vi "FPGA_SystemAsync VI Agent.vi"() -> ()   [LabVIEW 2017]
uses:
  <vilib>/Rock Robotics/SystemInterfaces/System/FPGA_SystemFPGA Ref Global.vi
panel:
  in  "Main Name":string
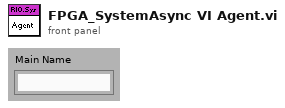
[diagram p1: front panel]
types:
  T1 = typedef "FPGA_SystemFRC FPGA Ref.ctl" = refnum<k20>
  T2 = enum32{"Bad", "Idle", "Run top level", "Running"}
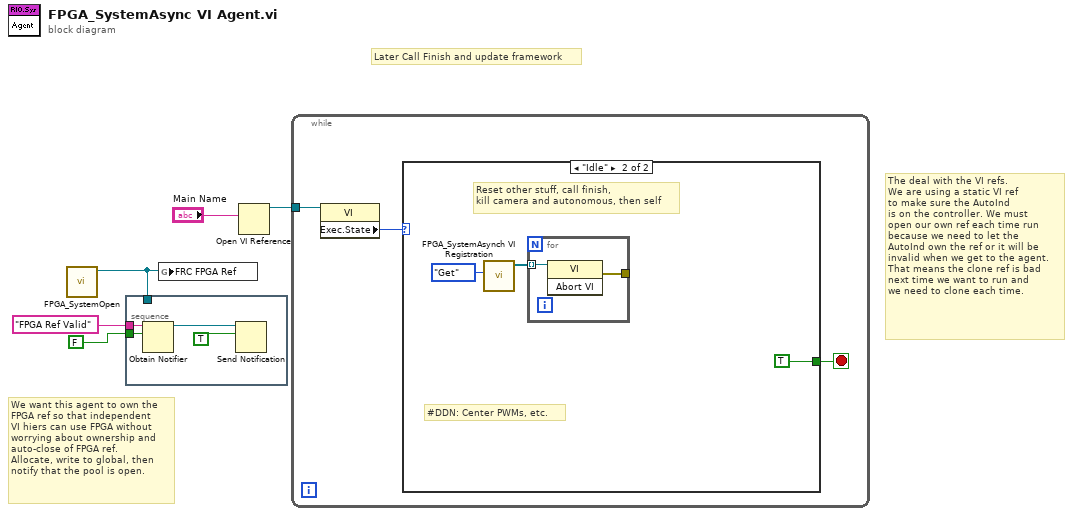
[diagram p0: block diagram]
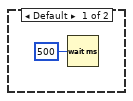
[diagram p2: hidden frame]
diagram:
  # "The deal with the VI refs.\nWe are using a static VI ref\nto make sure the AutoInd\nis on the controller. We must\nopen our own ref each time run\nbecause we need to let the\nAutoInd own the ref or it will be\ninvalid when we get to the agent.\nThat means the clone ref is bad\nnext time we want to run and\nwe need to clone each time."
  # "Later Call Finish and update framework"
  # "We want this agent to own the\nFPGA ref so that independent\nVI hiers can use FPGA without\nworrying about ownership and\nauto-close of FPGA ref.\nAllocate, write to global, then\nnotify that the pool is open."
  n1 = call <vilib>:"FPGA_SystemOpen.vi"() -> ("FRC FPGA Ref"=w1:T1)  [unwired: 11 out]
  n2 = stacked-sequence {
    tunnel: "FPGA Ref Valid" ("name (unnamed)") -> [w9]
    tunnel: FALSE -> [w8]
    tunnel: w1 -> [_]
    frame #0 {
      n3 = Obtain Notifier(name (unnamed)=w9, notification data type=w8) -> (notifier out=w7:refnum<notifier>)  [unwired: 2 in, 2 out]
      n4 = Send Notification(notification=TRUE, notifier=w7) -> ()  [unwired: 1 in, 2 out]
    }
  }
  n5 = global write "FPGA_SystemFPGA Ref Global.vi" "FRC FPGA Ref"(w1) -> ()
  n6 = Open VI Reference(vi path="Main Name") -> (vi reference=w4:refnum<vi>)  [unwired: 1 in, 5 out]
  n7 = while {
    tunnel: w4 -> [w10]
    stop <- w11 stop-if-true
    n8 = property class="VI"(reference=w10) -> ("Exec.State"=w12:T2)  [unwired: 1 in, 2 out]
    n9 = case shown="\"Idle\"" w12 {
      tunnel: [_ TRUE] -> w11
      frame Default {
        n10 = Wait (ms)(milliseconds to wait=u32 500) -> ()  [unwired: 1 out]
      }
      frame "Idle" {
        # "#DDN: Center PWMs, etc."
        # "Reset other stuff, call finish,\nkill camera and autonomous, then self"
        n11 = call <vilib>:"FPGA_SystemAsynch VI Registration.vi"("Operation"=enum16{"Get", "Add", "Remove"}."Get") -> ("VI Refs"=w15:refnum<vi>[])  [unwired: 1 in, 9 out]
        n12 = for {
          tunnel: w15 -> [w18] mode=indexing
          tunnel: [w17] -> _
          n13 = invoke class="VI" method="Abort VI"(reference=w18) -> (error out=w17:errorcluster)  [unwired: 2 in, 2 out]
        }
      }
    }
  }
